vi "Realease QHM.vi"(2 "error in (no error)":errorcluster, 3 "QHM in":refnum<queue>) -> (0 "error out":errorcluster)   [LabVIEW 2020, in "QHM.lvlib"]
uses:
  QHM.lvlib
  Type Defs/QMH Cluster.ctl
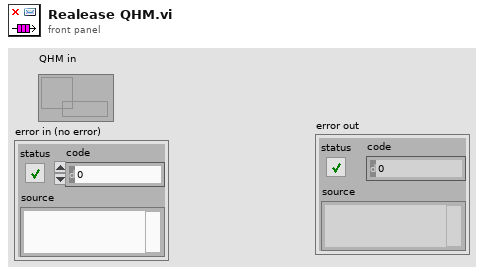
[diagram p1: front panel]
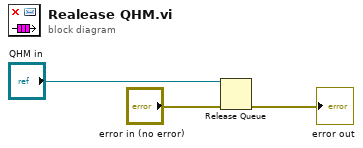
[diagram p0: block diagram]
diagram:
  n1 = Release Queue(queue="QHM in", error in (no error)="error in (no error)") -> (error out=→"error out":errorcluster)  [unwired: 1 in, 2 out]
